vi "ToneFit.vi"(6 "advanced search":T1={"approx freq. (optional)"=-1.0, "search (+/- % of Fsampl.)"=5.0} {"search (+/- % of Fsampl.)" format="%0.2p"; "approx freq. (optional)" format="%0.2p"}, 11 "Input data":dbl[](array[numeric])) -> (2 "Phase":dbl, 3 "Amplitude":dbl, 4 "XY Graph":cluster{"X-values":dbl[], "Input data":dbl[]}[](graph), 5 "Frequency":dbl)   [LabVIEW 2015]
uses:
  <vilib>/Analysis/coordinate.llb/Angle Units.ctl
  <vilib>/Analysis/coordinate.llb/Angle Range (Degree).ctl
  <vilib>/Analysis/coordinate.llb/Wrap Angle (scalar).vi
  <vilib>/measure/matone.llb/Extract Single Tone Information 1 Chan.vi
  <vilib>/Waveform/WDTOps.llb/WDT Get XY Value DBL.vi
  <vilib>/Analysis/NI_AAL_Angle.lvlib
  <vilib>/measure/NI_MAPro.lvlib
  <vilib>/Analysis/NI_AALPro.lvlib
panel:
  out "Slope":dbl
  in  "X-values":dbl[](array[numeric])
  out "Offset":dbl format="%0.2f"
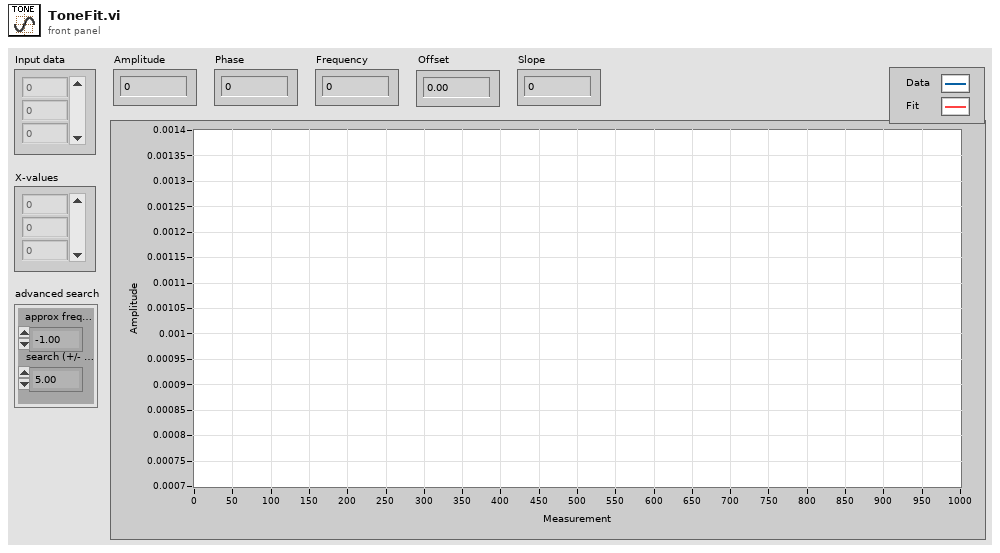
[diagram p1: front panel]
types:
  T1 = cluster{"approx freq. (optional)":dbl, "search (+/- % of Fsampl.)":dbl}
  T2 = enum32{"none", "input signal", "detected signal", "residual signal"}
  T3 = typedef "NI_AAL_Angle.lvlib/Angle Range (Degree).ctl" = u16
  T4 = typedef "NI_AAL_Angle.lvlib/Angle Units.ctl" = i32
  T5 = cluster{"exported time signal":waveform(dbl), "exported spectrum (dB)":cluster{"f0":dbl, "df":dbl, "dB Spectrum (Hann)":dbl[]}}
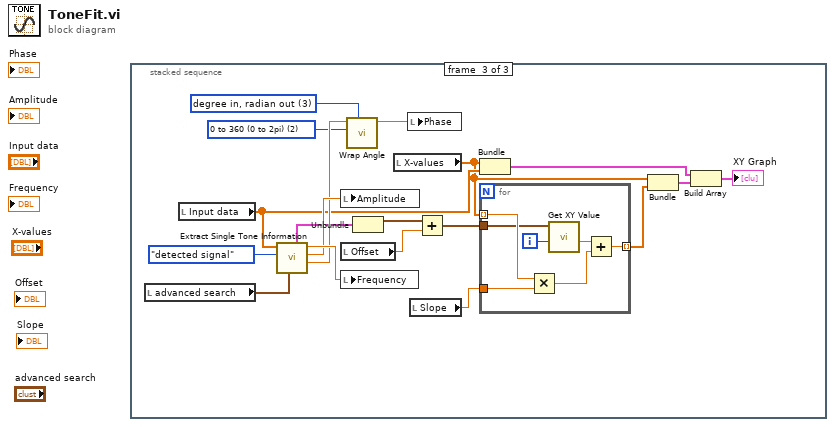
[diagram p0: block diagram]
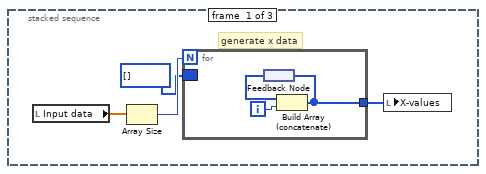
[diagram p2: hidden frame]
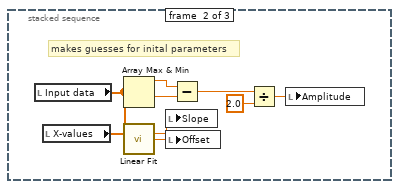
[diagram p3: hidden frame]
diagram:
  n1 = stacked-sequence {
    frame #0 {
      # "generate x data"
      n2 = local read "Input data"() -> (w2:dbl[])
      n3 = Array Size(array=w2) -> (size(s)=w4:i32)
      n4 = for {
        N: w4 -> [_]
        border: i32[] [] -> [_]
        tunnel: [w5] -> w1
        i -> [w6]
        n5 = feedback #1() -> (w7:i32[])
        n6 = Build Array (concatenate)(w7, w6) -> (w5:i32[])
        n7 = feedback-in #1(w5) -> ()
      }
      n8 = local write "X-values"(w1) -> ()
    }
    frame #1 {
      # "makes guesses for inital parameters"
      n9 = local read "Input data"() -> (w9:dbl[])
      n10 = local read "X-values"() -> (w11:dbl[])
      n11 = Array Max & Min(array=w9) -> (max value=w15:dbl, min value=w16:dbl)  [unwired: 2 out]
      n12 = call <vilib>:"Linear Fit.vi"("Y"=w9, "X"=w11) -> ("slope"=w10:dbl, "intercept"=w8:dbl)  [unwired: 9 in, 3 out]
      n13 = local write "Slope"(w10) -> ()
      n14 = local write "Offset"(w8) -> ()
      n15 = Subtract(x=w15, y=w16) -> (x-y=w14:dbl)
      n16 = Divide(x=w14, y=2.0) -> (x/y=w12:dbl)
      n17 = local write "Amplitude"(w12) -> ()
    }
    frame #2 {
      w30 = T3 2 items=["none", "-180 to 180 (-pi to pi)", "0 to 360 (0 to 2pi)"] ("angle range")
      w31 = T4 3 items=["radian in, radian out", "radian in, degree out", "degree in, degree out", "degree in, radian out"] ("angle units")
      n18 = local read "advanced search"() -> (w29:T1)
      n19 = local read "Input data"() -> (w25:dbl[])
      n20 = call-poly <vilib>:"Extract Single Tone Information.vi"("advanced search"=w29, "export mode"=T2."detected signal", "time signal in"=w25) -> ("detected phase (deg)"=w33:dbl, "detected amplitude"=w34:dbl, "detected frequency"=w35:dbl, "exported signals"=w28:T5)  [unwired: 3 in, 2 out]
      n21 = local write "Amplitude"(w34) -> ()
      n22 = local read "Offset"() -> (w27:dbl)
      n23 = local write "Frequency"(w35) -> ()
      n24 = call-poly <vilib>:"Wrap Angle.vi"("angle units"=w31, "angle range"=w30, "angle in"=w33) -> ("angle out"=w32:dbl)  [unwired: 7 in, 1 out]
      n25 = Unbundle(w28) -> ("exported time signal"=w24:waveform(dbl))  [unwired: 1 out]
      n26 = local read "X-values"() -> (w20:dbl[])
      n27 = local write "Phase"(w32) -> ()
      n28 = local read "Slope"() -> (w26:dbl)
      n29 = Add(x=w24, y=w27) -> (x+y=w22:waveform(dbl))
      n30 = Bundle("X-values"=w20, "Input data"=w25) -> (w19:cluster{"X-values":dbl[], "Input data":dbl[]})  [unwired: 1 in]
      n31 = for {
        tunnel: w26 -> [w42]
        tunnel: w20 -> [w41] mode=indexing
        tunnel: [w39] -> w21 mode=indexing
        tunnel: w22 -> [w38]
        i -> [w37]
        n32 = Multiply(x=w41, y=w42) -> (x*y=w40:dbl)
        n33 = call-poly <vilib>:"Get XY Value.vi"("Y position"=w37, "waveform in"=w38) -> ("Y value"=w36:dbl)  [unwired: 5 in, 4 out]
        n34 = Add(x=w36, y=w40) -> (x+y=w39:dbl)
      }
      n35 = Bundle("X-values"=w20, w21) -> (w18:cluster{"X-values":dbl[], dbl[]})  [unwired: 1 in]
      n36 = Build Array(w19, w18) -> (→"XY Graph":cluster{"X-values":dbl[], "Input data":dbl[]}[])
    }
  }
